vi "philtec_ui.vi"() -> ()   [LabVIEW 2012]
doc: "I. Description:\nThis example demonstrates how to acquire a continuous amount of data (Waveform) using the DAQ device's internal clock.\n\nII. Instructions for Running:\n1. Select the physical channel to correspond to where your signal is input on the DAQ device.\n2. Enter the minimum and maximum voltages.\nNote: For better accuracy try to match the input range to the expected voltage level of the measured signal.\n3. Select the number of samples to acquire per loop iteration.\n4. Set the rate of the acquisition\nNote: The rate should be AT LEAST twice as fast as the maximum frequency component of the signal being acquired.\n\nIII. Block Diagram Steps:\n1. Create an analog input voltage channel.\n2. Set the rate for the sample clock. Additionally, define the sample mode to be continuous.\n3. Call the Start VI to start the acquisition.\n4. Read the waveform data in a loop until the user hits the stop button or an error occurs.\nNote: This example reads data from one or more channels and returns an array of data. Use the Index Array function to access an individual channel of data.\n5. Call the Clear Task VI to clear the Task.\n6. Use the popup dialog box to display an error if any.\n\nIV. I/O Connections Overview:\nMake sure your signal input terminal matches the Physical Channel I/O Control. For further connection information, refer to your hardware reference manual."
uses:
  <vilib>/Utility/error.llb/DialogType.ctl
  <vilib>/DAQmx/read.llb/DAQmx Read (Analog Wfm 1Chan NSamp).vi
  <vilib>/DAQmx/create/channels.llb/DAQmx Create Channel (AI-Voltage-Basic).vi
  <vilib>/DAQmx/configure/timing.llb/DAQmx Timing (Sample Clock).vi
  <vilib>/Analysis/2dsp.llb/Decimate (single shot, DBL).vi
  <vilib>/DAQmx/miscellaneous.llb/DAQmx Fill In Error Info.vi
  <vilib>/Analysis/NI_AALPro.lvlib
panel:
  out "um RMS":dbl format="%#.2f"
  in  "Run":bool
  in  "Restart Averaging":bool
  out "Spectrum":cluster{"X out":dbl[], dbl[]}[](graph)
  in  "N points":u32=30
  in  "Frequency range":cluster{"Min":dbl, "Max":dbl}={"Min"=10.0, "Max"=250.0} {"Max" format="%#_3p"; "Min" format="%#_3p"}
  in  "Integrator scaling":bool
  in  "Window":T1(ring)
  in  "Averaging Parameters":T2={"averaging mode"=0, "weighting mode"=1, "number of averages"=10} {"averaging mode" items=["No averaging", "Vector averaging", "RMS averaging", "Peak hold"]; "weighting mode" items=["Linear", "Exponential"]}
  in  "Run":bool
  in  "Chart decimate":i32=10
  out "Log":waveform(dbl)(graph)
  out "Position":dbl format="%#.2f"
  out "Calibration (um/V)":dbl=384.63406259495224
  in  "Zero":bool
  in  "Calibrate":bool
  out "Raw voltage":dbl
  in  "Decimate":i32=100
  in  "Length (sec)":dbl=2.0
  in  "Physical Channel":tag="Dev1/ai0"
  in  "Minimum Value":dbl=-10.0 format="%0.2f"
  in  "Maximum Value":dbl=10.0 format="%0.2f"
  in  "stop":bool
  in  "Sample Rate":dbl=50000.0 caption="Sample Rate (Hz)" format="%.2p"
  out "HF signal":waveform(dbl)(graph)
  # "Channel Parameters"
  # "Timing Parameters"
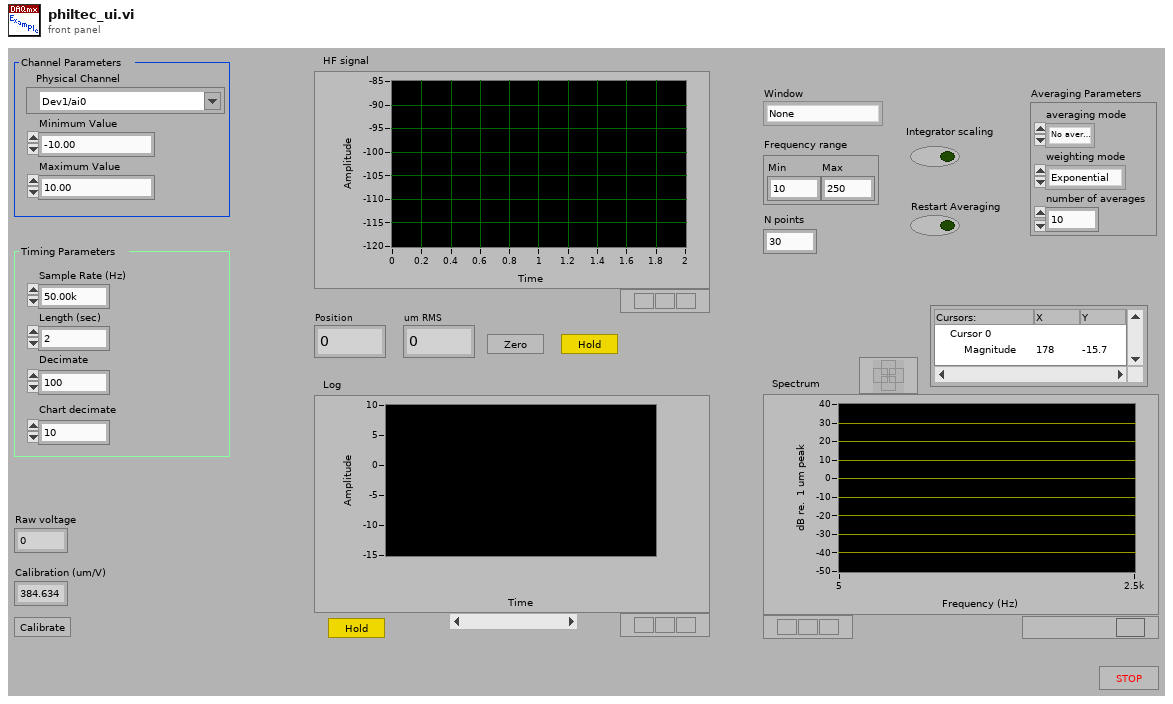
[diagram p1: front panel]
types:
  T1 = enum16{"None ", "Hanning", "Hamming", "Blackman-Harris", "Exact Blackman", "Blackman", "Flat Top", "4 Term B-Harris ", "7 Term B-Harris", "Low Sidelobe"}
  T2 = cluster{"averaging mode":u16, "weighting mode":u16, "number of averages":u32}
  T3 = typedef "DialogType.ctl" = u16
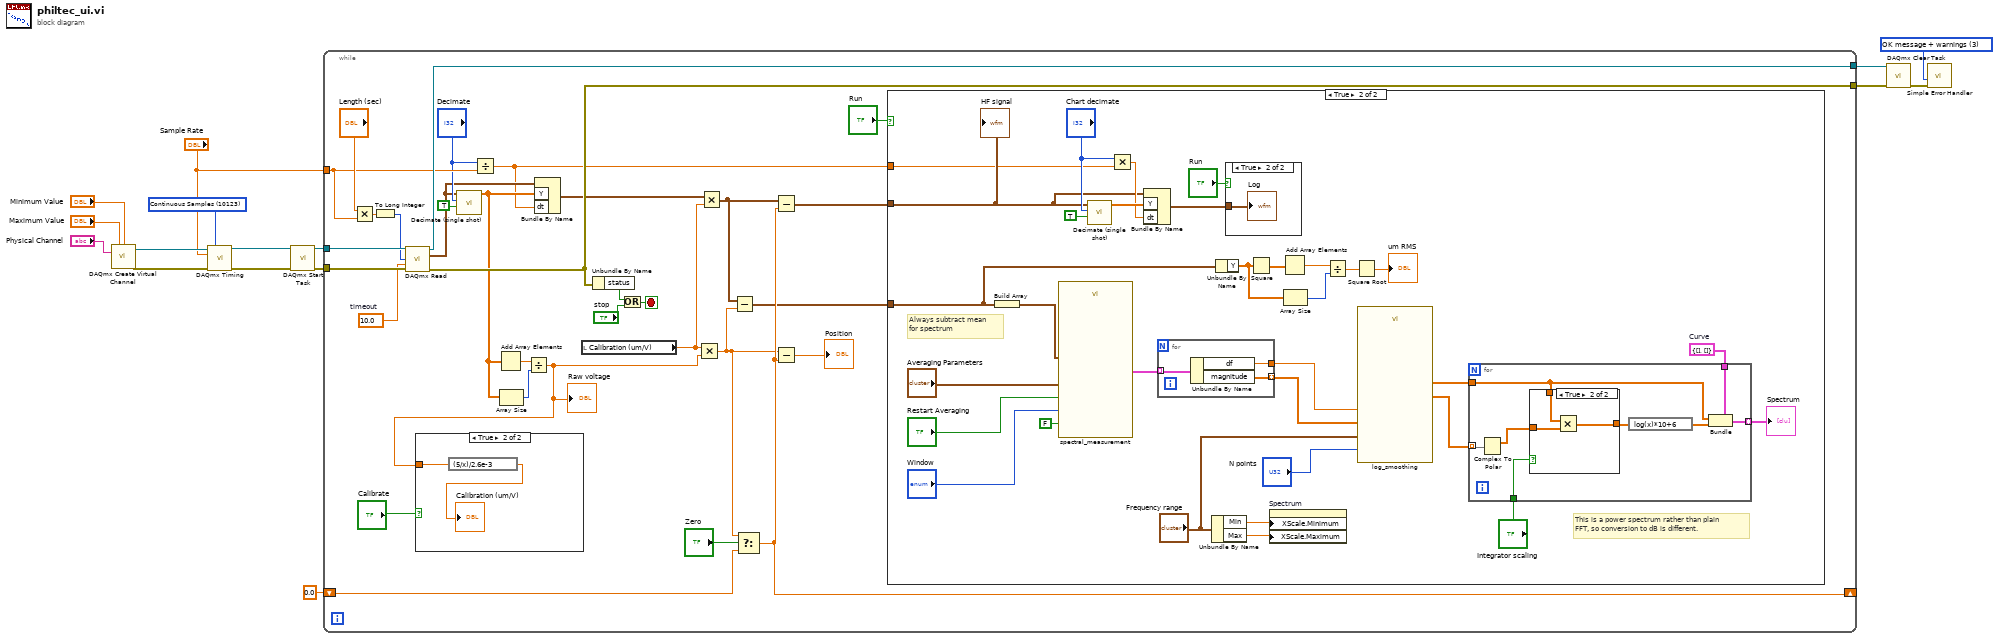
[diagram p0: block diagram]
diagram:
  w3 = T3 3 items=["no dialog", "OK message", "continue or stop message", "OK message + warnings", "continue/stop + warnings"] ("type of dialog (OK msg:1)")
  w7 = 10123 items=["Finite Samples"=10178, "Continuous Samples"=10123] ("sample mode")
  n1 = call-poly <vilib>:"DAQmx Create Virtual Channel.vi"("maximum value"="Maximum Value", "minimum value"="Minimum Value", "physical channels"="Physical Channel") -> ("task out"=w11:refnum<k21>, "error out"=w14:errorcluster)  [unwired: 11 in]
  n2 = call-poly <vilib>:"DAQmx Timing.vi"("task/channels in"=w11, "sample mode"=w7, "rate"="Sample Rate", "error in"=w14) -> ("task out"=w6:refnum<k21>, "error out"=w5:errorcluster)  [unwired: 10 in]
  n3 = call <vilib>:"DAQmx Start Task.vi"("task/channels in"=w6, "error in"=w5) -> ("task out"=w10:refnum<k21>, "error out"=w13:errorcluster)  [unwired: 12 in]
  n4 = while {
    tunnel: w13 -> [w48]
    tunnel: w10 -> [w47]
    tunnel: [w46] -> w9
    tunnel: [w45] -> w4
    tunnel: "Sample Rate" -> [w34]
    shift-right: [w26] -> _
    shift-left: 0.0 ("x*y") -> [w30]
    stop <- w43 stop-if-true
    w41 = 10.0  # timeout
    n5 = Multiply(x="Length (sec)", y=w34) -> (x*y=w37:dbl)
    n6 = To Long Integer(number=w37) -> (32bit integer=w35:i32)
    n7 = call-poly <vilib>:"DAQmx Read.vi"("task/channels in"=w47, "number of samples per channel"=w35, "timeout"=w41, "error in"=w48) -> ("task out"=w46:refnum<k21>, "data"=w24:waveform(dbl), "error out"=w45:errorcluster)  [unwired: 9 in]
    n8 = call-poly <vilib>:"Decimate (single shot).vi"("averaging"=TRUE, "decimating factor"="Decimate", "X"=w24) -> ("Decimated Array"=w25:dbl[])  [unwired: 7 in, 1 out]
    n9 = Divide(x="Decimate", y=w34) -> (x/y=w19:dbl)
    n10 = Add Array Elements(numeric array=w25) -> (sum=w39:dbl)
    n11 = Array Size(array=w25) -> (size(s)=w38:i32)
    n12 = Divide(x=w39, y=w38) -> (x/y=w31:dbl)
    "Raw voltage" <- w31
    n13 = case shown="True" "Calibrate" {
      tunnel: w31 -> [_ w98]
      frame False {
      }
      frame True {
        n14 = expression code="(5/x)/2.6e-3"(w98) -> (→"Calibration (um/V)":dbl)
      }
    }
    n15 = Bundle By Name(cluster=w24, "Y"=w25, "dt"=w19) -> (w18:waveform(dbl))
    n16 = local read "Calibration (um/V)"() -> (w27:dbl)
    n17 = Unbundle By Name(w45) -> ("status"=w44:bool)
    n18 = Or(x=w44, y="stop") -> (x .or. y?=w43:bool)
    n19 = Multiply(x=w27, y=w31) -> (x*y=w20:dbl)
    n20 = Multiply(x=w18, y=w27) -> (x*y=w21:waveform(dbl))
    n21 = Subtract(x=w21, y=w20) -> (x-y=w22:waveform(dbl))
    n22 = Select(t=w20, s="Zero", f=w30) -> (s? t:f=w26:dbl)
    n23 = Subtract(x=w21, y=w26) -> (x-y=w23:waveform(dbl))
    n24 = Subtract(x=w20, y=w26) -> (x-y=→"Position":dbl)
    n25 = case shown="True" "Run" {
      tunnel: w23 -> [_ w57]
      tunnel: w22 -> [_ w55]
      tunnel: w19 -> [_ w56]
      frame False {
      }
      frame True {
        w70 = cluster{"X":dbl[], "Y":dbl[]} {"X"=[], "Y"=[]}  # Curve
        # "This is a power spectrum rather than plain\nFFT, so conversion to dB is different."
        # "Always subtract mean \nfor spectrum"
        n26 = Build Array(w55) -> (w58:waveform(dbl)[])
        n27 = call "spectral_measurement.vi"("Signals"=w58, "Restart Averaging"="Restart Averaging", "dB On"=FALSE, "Spectrum Averaging Parameters"="Averaging Parameters", "Window"="Window") -> ("PSD"=w72:cluster{"f0":dbl, "df":dbl, "magnitude":dbl[]}[])  [unwired: 8 in, 2 out]
        n28 = call-poly <vilib>:"Decimate (single shot).vi"("averaging"=TRUE, "decimating factor"="Chart decimate", "X"=w57) -> ("Decimated Array"=w79:dbl[])  [unwired: 7 in, 1 out]
        n29 = Multiply(x="Chart decimate", y=w56) -> (x*y=w78:dbl)
        n30 = Bundle By Name(cluster=w57, "Y"=w79, "dt"=w78) -> (w76:waveform(dbl))
        n31 = for {
          tunnel: w72 -> [w83] mode=indexing
          tunnel: [w82] -> w69
          tunnel: [w81] -> w71 mode=indexing
          n32 = Unbundle By Name(w83) -> ("df"=w82:dbl, "magnitude"=w81:dbl[])
        }
        n33 = Unbundle By Name("Frequency range") -> ("Min"=w63:dbl, "Max"=w62:dbl)
        n34 = Unbundle By Name(w55) -> ("Y"=w53:dbl[])
        n35 = case shown="True" "Run" {
          tunnel: w76 -> [_ w96]
          frame False {
          }
          frame True {
            "Log" <- w96
          }
        }
        n36 = Square(x=w53) -> (x^2=w54:dbl[])
        n37 = property on="Spectrum" class="XYGraph (strict)"("XScale.Minimum"=w63, "XScale.Maximum"=w62) -> ()  [unwired: 2 in, 2 out]
        n38 = Add Array Elements(numeric array=w54) -> (sum=w52:dbl)
        n39 = Array Size(array=w53) -> (size(s)=w51:i32)
        n40 = Divide(x=w52, y=w51) -> (x/y=w50:dbl)
        n41 = Square Root(x=w50) -> (sqrt(x)=→"um RMS":dbl)
        n42 = call "log_smoothing.vi"("N points"="N points", "Y"=w71, "Frequency range"="Frequency range", "Frequency resolution (Hz)"=w69) -> ("Y out"=w66:cdb[][], "X out"=w67:dbl[])  [unwired: 6 in]
        n43 = for {
          tunnel: w66 -> [w91] mode=indexing
          tunnel: w67 -> [w85]
          tunnel: [w90] -> w68 mode=indexing
          tunnel: "Integrator scaling" -> [w86]
          tunnel: w70 -> [w84]
          n44 = Complex To Polar(r * e^(i*theta)=w91) -> (r=w87:dbl[])  [unwired: 1 out]
          n45 = case shown="True" w86 {
            tunnel: [w92 w93] -> w88
            tunnel: w87 -> [w92 w95]
            tunnel: w85 -> [_ w94]
            frame False {
            }
            frame True {
              n46 = Multiply(x=w94, y=w95) -> (x*y=w93:dbl[])
            }
          }
          n47 = expression code="log(x)*10+6"(w88) -> (w89:dbl[])
          n48 = Bundle(cluster=w84, "X"=w85, "Y"=w89) -> (w90:cluster{"X":dbl[], "Y":dbl[]})
        }
        "Spectrum" <- w68
        "HF signal" <- w57
      }
    }
  }
  n49 = call <vilib>:"DAQmx Clear Task.vi"("task in"=w9, "error in"=w4) -> ("error out"=w12:errorcluster)  [unwired: 13 in]
  n50 = call <vilib>:"Simple Error Handler.vi"("type of dialog (OK msg:1)"=w3, "error in (no error)"=w12) -> ()  [unwired: 3 in, 5 out]
